vi "Test_Calculate Drop-out.vi"(8 "V_MIN":dbl, 9 "Amps":T2 format="%5.3f A", 10 "Volts":T1 format="%5.3f V", 11 "Table in":refnum<vi>) -> ()   [LabVIEW 2025]
uses:
  Controls/Numeric Current.ctl
  Controls/Numeric Voltage.ctl
panel:
  out "concatenated string":string
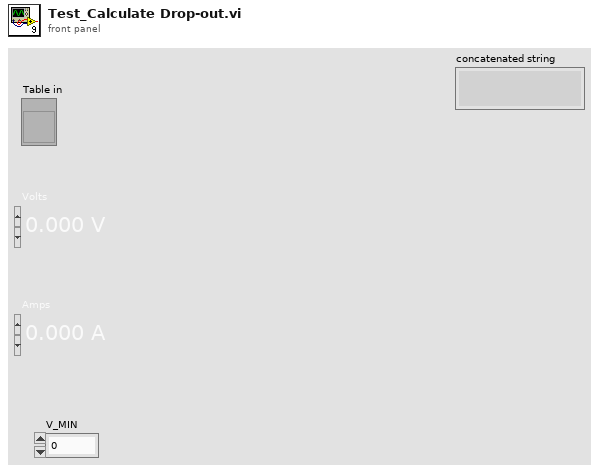
[diagram p1: front panel]
types:
  T1 = typedef "Numeric Voltage.ctl" = dbl
  T2 = typedef "Numeric Current.ctl" = dbl
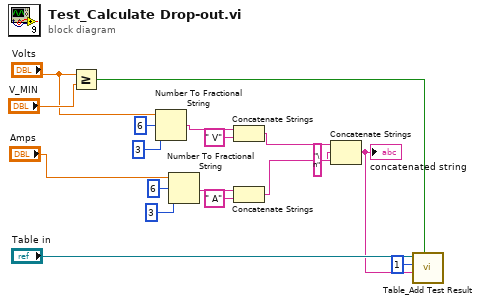
[diagram p0: block diagram]
diagram:
  n1 = Greater Or Equal?(x="Volts", y="V_MIN") -> (x >= y?=w16:bool)
  n2 = Number To Fractional String(number="Volts", width (-)=i16 6, precision (6)=i16 3) -> (F-format string=w9:string)  [unwired: 1 in]
  n3 = Number To Fractional String(number="Amps", width (-)=i16 6, precision (6)=i16 3) -> (F-format string=w6:string)  [unwired: 1 in]
  n4 = Concatenate Strings(w9, " V" ("string")) -> (w5:string)
  n5 = Concatenate Strings(w6, " A" ("string")) -> (w4:string)
  n6 = Concatenate Strings(w5, "\n" ("string"), w4) -> (w2:string)
  "concatenated string" <- w2
  n7 = call "Table_Add Test Result.vi"("Pass?"=w16, "Test Result"=w2, "index (row)"=1, "Table in"="Table in") -> ()  [unwired: 7 in, 1 out]
